vi "Expand Pin Groups and Identify Pin Types.vi"(0 "TSM context":T4, 5 "Pins and/or Pin Groups":tag[](array[tag]), 11 "error in":errorcluster) -> (4 "Pins and/or Pin Groups Information":T3[](array[typedef]), 6 "Expanded Pin Information":T1[](array[typedef]), 15 "error out":errorcluster)   [LabVIEW 2020]
uses:
  <vilib>/NI_TestStand_SemiconductorModule/NI_TestStand_Semiconductor_Module.lvlibp/PinMap/General/SemiconductorModuleContext.ctl
  TSM Pin Information.ctl
  TSM Pin Type Identifier.ctl
  TSM Expanded Pin Information.ctl
  <vilib>/NI_TestStand_SemiconductorModule/NI_TestStand_Semiconductor_Module.lvlibp/PinMap/Advanced/GetPinsInPinGroup.vi
  <vilib>/NI_TestStand_SemiconductorModule/NI_TestStand_Semiconductor_Module.lvlibp
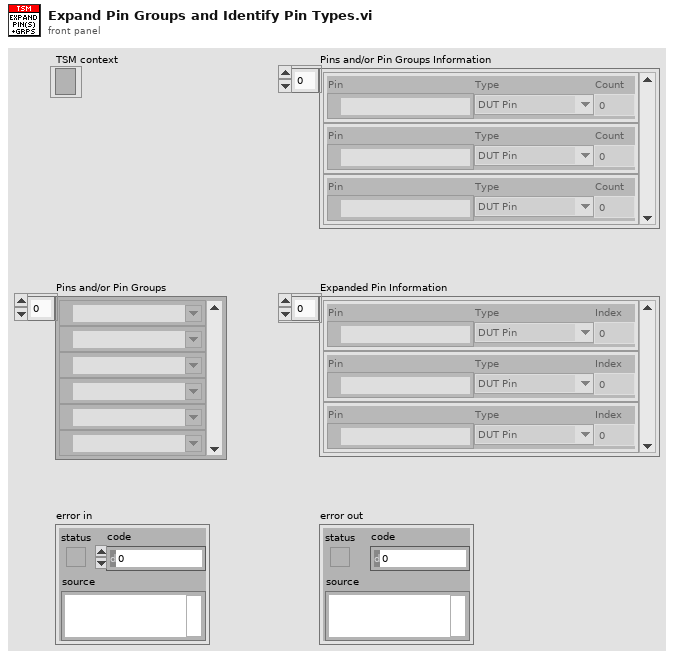
[diagram p1: front panel]
types:
  T1 = typedef "TSM Expanded Pin Information.ctl" = cluster{"Pin":tag, "Type":T2, "Index":i32}
  T2 = typedef "TSM Pin Type Identifier.ctl" = enum8{"DUT Pin", "System Pin", "Pin Group", "Not Determined"}
  T3 = typedef "TSM Pin Information.ctl" = cluster{"Pin":tag, "Type":T2, "Count":i32}
  T4 = typedef "NI_TestStand_Semiconductor_Module.lvlibp/SemiconductorModuleContext.ctl" = refnum<k7>
  T5 = typedef "NI_TestStand_Semiconductor_Module.lvlibp/TSM_Pin.ctl" = tag
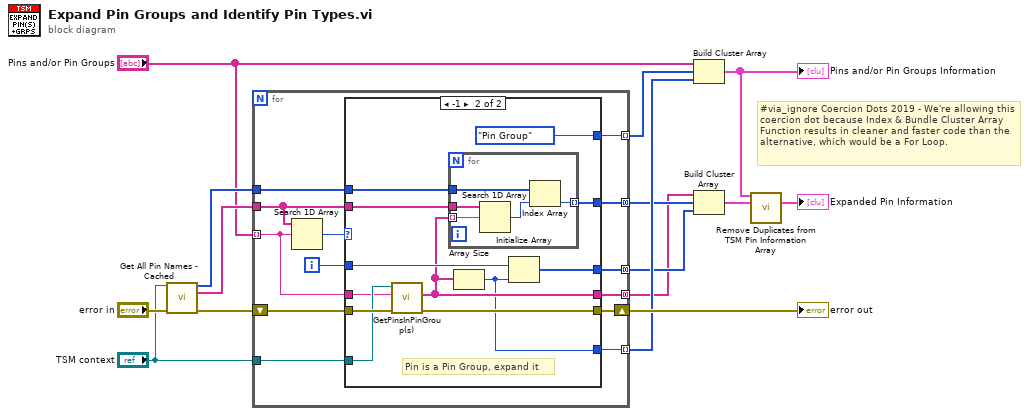
[diagram p0: block diagram]
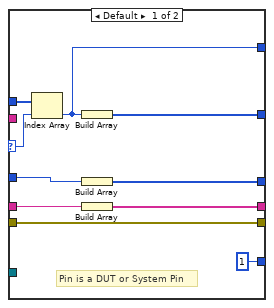
[diagram p2: hidden frame]
diagram:
  # "#via_ignore Coercion Dots 2019 - We're allowing this coercion dot because Index & Bundle Cluster Array Function results in cleaner and faster code than the alternative, which would be a For Loop."
  n1 = call "Get All Pin Names - Cached.vi"("TSM Context in"="TSM context", "error in"="error in") -> ("Pin Types"=w11:T2[], "Pin Names"=w10:tag[], "error out"=w13:errorcluster)  [unwired: 11 in]
  n2 = for {
    shift-right: [w28] -> w15
    shift-left: w13 -> [w27]
    tunnel: "Pins and/or Pin Groups" -> [w24] mode=indexing
    tunnel: [w25] -> w8 mode=indexing
    tunnel: [w21] -> w5 mode=concatenating
    tunnel: [w23] -> w4 mode=concatenating
    tunnel: "TSM context" -> [w20]
    tunnel: [w19] -> w6 mode=concatenating
    tunnel: w11 -> [w18]
    tunnel: w10 -> [w17]
    tunnel: [w16] -> w7 mode=indexing
    i -> [w22]
    n3 = Search 1D Array(1D array=w17, element=w24) -> (index of element=w26:i32)  [unwired: 1 in]
    n4 = case shown="-1" w26 {
      selector: w26 -> [w36 _]
      tunnel: [w38 w50] -> w28
      tunnel: w27 -> [w38 w49]
      tunnel: w18 -> [w37 w41]
      tunnel: [w31 TSM_Pin_Type_Identifier."Pin Group" ("Enum")] -> w25
      tunnel: w24 -> [w35 w47]
      tunnel: [w34 w43] -> w23
      tunnel: w22 -> [w33 w46]
      tunnel: [w32 w45] -> w21
      tunnel: w20 -> [_ w48]
      tunnel: w17 -> [_ w42]
      tunnel: [w30 w40] -> w19
      tunnel: [1 w39] -> w16
      frame Default {
        # "Pin is a DUT or System Pin"
        n5 = Index Array(array=w37, index=w36) -> (element=w31:T2)
        n6 = Build Array(w31) -> (w30:T2[])
        n7 = Build Array(w33) -> (w32:i32[])
        n8 = Build Array(w35) -> (w34:tag[])
      }
      frame -1 {
        # "Pin is a Pin Group, expand it"
        n9 = call-poly <vilib>:"GetPinsInPinGroup(s).vi"("error in (no error)"=w49, "Pin Group"=w47, "Semiconductor Module Context"=w48) -> ("error out"=w50:errorcluster, "Pins"=w43:T5[])  [unwired: 6 in, 1 out]
        n10 = for {
          tunnel: w43 -> [w55] mode=indexing
          tunnel: w42 -> [w54]
          tunnel: w41 -> [w53]
          tunnel: [w51] -> w40 mode=indexing
          n11 = Search 1D Array(1D array=w54, element=w55) -> (index of element=w52:i32)  [unwired: 1 in]
          n12 = Index Array(array=w53, index=w52) -> (element=w51:T2)
        }
        n13 = Array Size(array=w43) -> (size(s)=w39:i32)
        n14 = Initialize Array(w46, w39) -> (w45:i32[])
      }
    }
  }
  "error out" <- w15
  n15 = Build Cluster Array("Pins and/or Pin Groups", w8, w7) -> (w2:cluster{"Pin":tag, "Enum":T2, i32}[])
  "Pins and/or Pin Groups Information" <- w2
  n16 = Build Cluster Array(w4, w6, w5) -> (w3:cluster{"Pin":T5, "Enum":T2, i32}[])
  n17 = call "Remove Duplicates from TSM Pin Information Array.vi"("Pins and/or Pin Groups Information"=w2, "Expanded Pin Information in"=w3) -> ("De-Duped Expanded Pin Information out"=→"Expanded Pin Information":T1[])  [unwired: 13 in]
